vi "根据信息获得棋子图片.vi"(1 "棋子颜色":enum16{"银色", "黑色"}(ring), 2 "背景颜色":enum16{"白色", "绿色"}(ring), 3 "棋子类型":enum16{"士兵", "骑士", "主教", "战车", "皇后", "国王", "空"}(ring)) -> (0 "棋子":u16(ring))   [LabVIEW 2017]
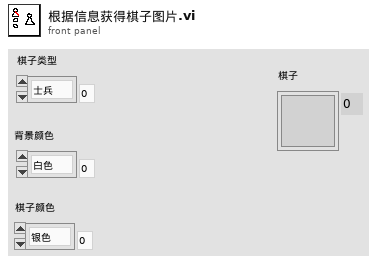
[diagram p1: front panel]
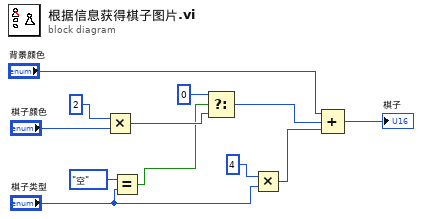
[diagram p0: block diagram]
diagram:
  n1 = Multiply(x=2, y="棋子颜色") -> (x*y=w11:i32)
  n2 = Equal?(x=enum16{"士兵", "骑士", "主教", "战车", "皇后", "国王", "空"}."空", y="棋子类型") -> (x = y?=w9:bool)
  n3 = Select(t=u16 0, s=w9, f=w11) -> (s? t:f=w6:i32)
  n4 = Multiply(x=4, y="棋子类型") -> (x*y=w7:i32)
  n5 = Compound Arithmetic op=ADD("背景颜色", w6, w7) -> (→"棋子":i32)
